vi "ShowString.vi"(8 "error in (no error)":errorcluster, 9 "SubQueueIN":refnum<queue>, 10 "MainQueueIN":refnum<queue>, 11 "Data Value Reference out":refnum<data-value>) -> (0 "error out":errorcluster, 3 "Data Value Reference out":refnum<data-value>)   [LabVIEW 2013]
uses:
  Control/SystemData.ctl
  Control/SignalType.ctl
  Control/SystemCommand.ctl
  Control/SubDaqCommand.ctl
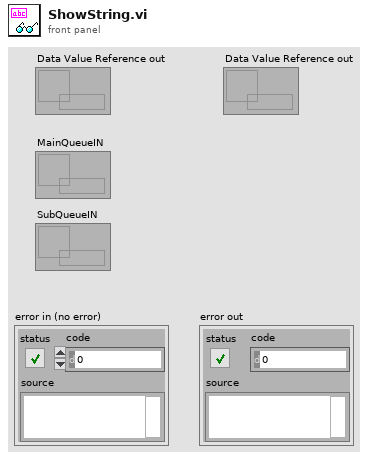
[diagram p1: front panel]
types:
  T1 = typedef "SystemData.ctl" = cluster{"Numeric":dbl, "String":string, "Boolean":bool, "Frequency":dbl, "Amplitude":dbl, "SignalType":T2, "WaveformArray":waveform(dbl)[], "Reset":bool, "StateString":string, "FFTmagnitudes":cluster{"f0":dbl, "df":dbl, "magnitude":dbl[]}[]}
  T2 = typedef "SignalType.ctl" = enum16{"Sin", "Triangle", "Square"}
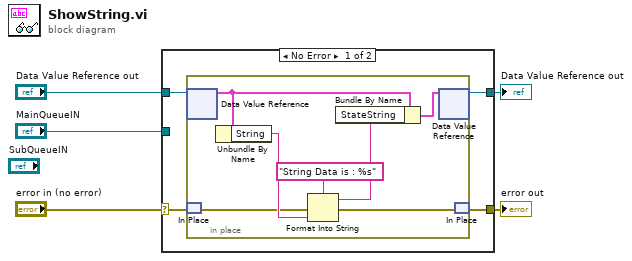
[diagram p0: block diagram]
diagram:
  n1 = case shown="No Error" "error in (no error)" {
    selector: "error in (no error)" -> [w8 w17]
    tunnel: "Data Value Reference out" -> [w9 w18]
    tunnel: [w7 w17] -> w2
    tunnel: "MainQueueIN" -> [_ _]
    tunnel: [w6 w18] -> w5
    frame No Error {
      n2 = in-place {
        n3 = in-place-dvr #1(w9) -> (w11:T1)  [unwired: 1 out]
        n4 = in-place-match #2(w8) -> (w14:errorcluster)
        n5 = Unbundle By Name(w11) -> ("String"=w16:string)
        n6 = Format Into String(format string="String Data is : %s", error in=w14, w16) -> (resulting string=w12:string, error out=w13:errorcluster)  [unwired: 1 in]
        n7 = Bundle By Name(cluster=w11, "StateString"=w12) -> (w10:T1)
        n8 = in-place-dvr #1(w10) -> (w6:refnum<data-value>)  [unwired: 1 out]
        n9 = in-place-match #2(w13) -> (w7:errorcluster)
      }
    }
    frame Error {
    }
  }
  "Data Value Reference out" <- w5
  "error out" <- w2
